vi "SaveQueue.vi"(0 "Program Interface in":refnum<class "Program Interface.lvclass">, 5 "error in (no error)":errorcluster) -> (14 "Program Interface out":refnum<class "Program Interface.lvclass">, 19 "error out":errorcluster)   [LabVIEW 2019, in "Program Interface.lvclass"]
uses:
  Program Interface.lvclass
  Program Interface.lvclass/Program Interface.ctl
  SavedQueue.ctl
  <vilib>/Utility/file.llb/Write Delimited Spreadsheet (string).vi
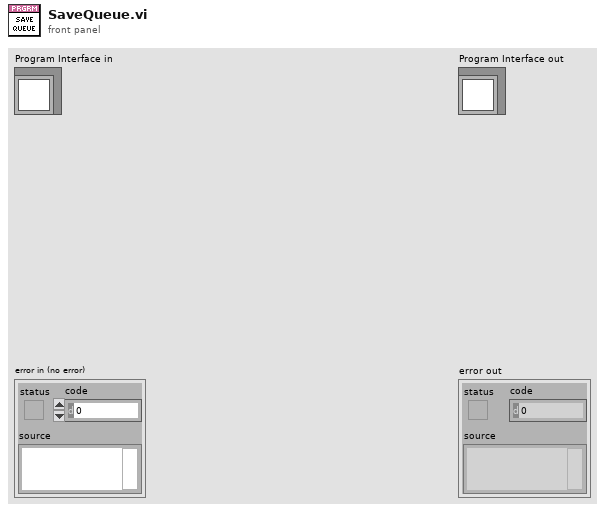
[diagram p1: front panel]
types:
  T1 = typedef "Program Interface.lvclass/SavedQueue.ctl" = cluster{"Name":string, "Programs":string[]}
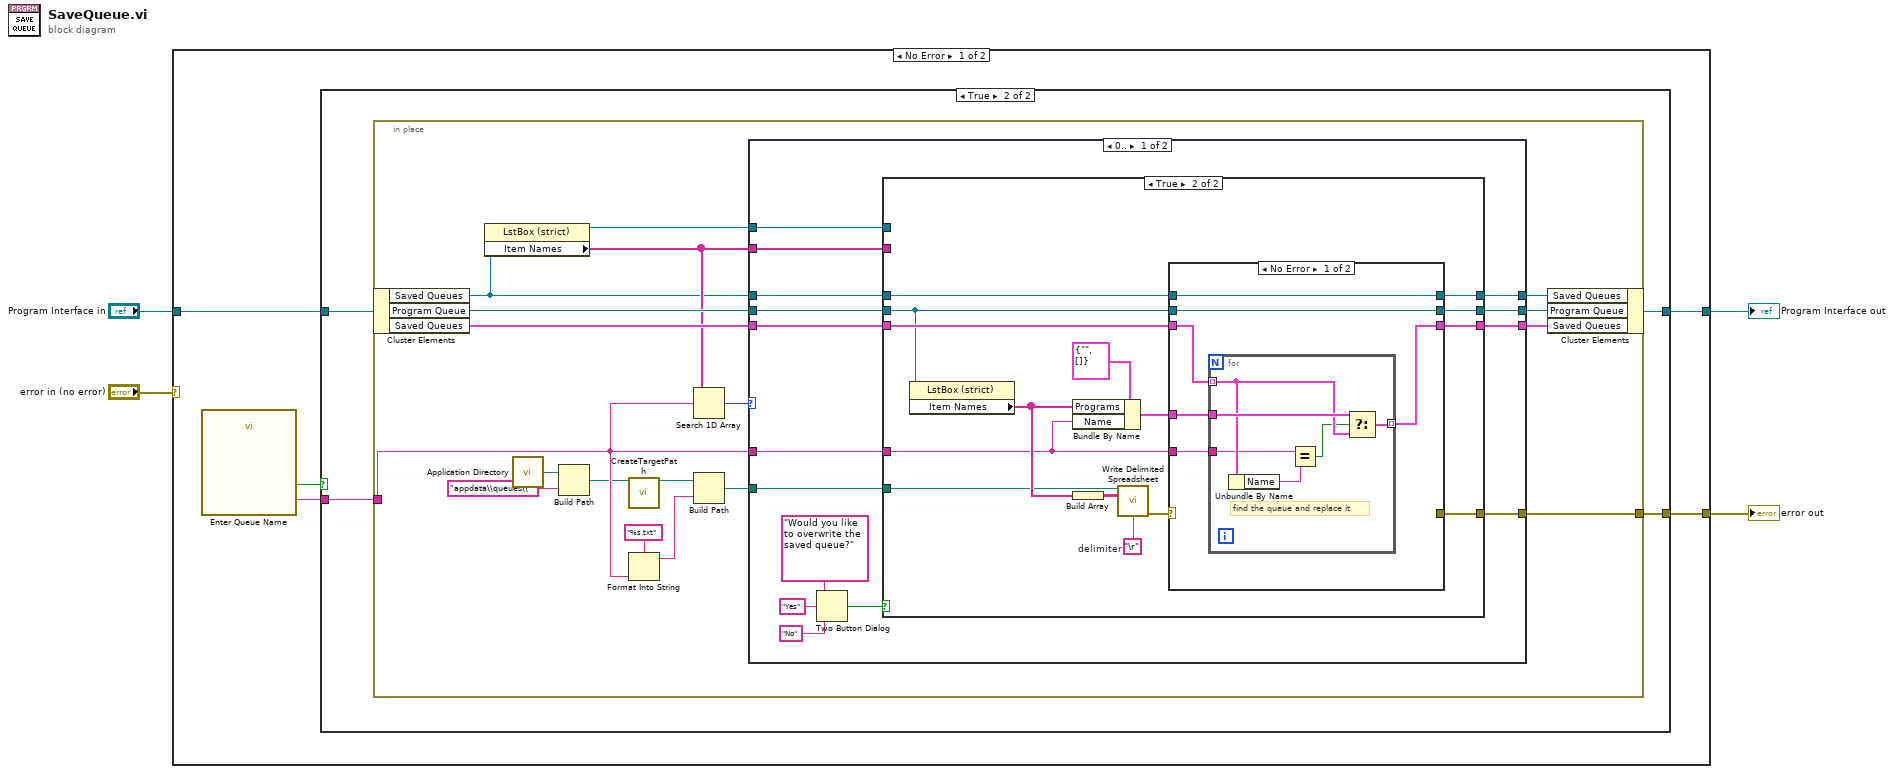
[diagram p0: block diagram]
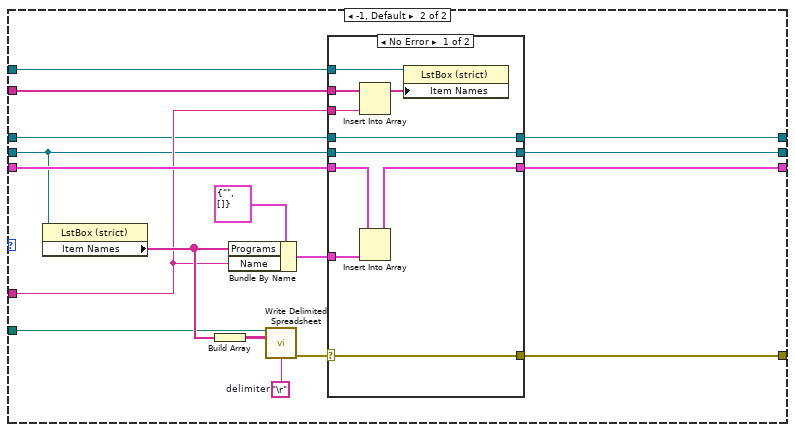
[diagram p5: hidden frame]
diagram:
  n1 = case shown="No Error" "error in (no error)" {
    selector: "error in (no error)" -> [_ w114]
    tunnel: [w9 w114] -> w3
    tunnel: [w7 w113] -> w1
    tunnel: "Program Interface in" -> [w8 w113]
    frame No Error {
      n2 = call "Enter Queue Name"() -> ("Queue Name"=w6:string, "OK"=w5:bool)  [unwired: 17 in, 1 out]
      n3 = case shown="True" w5 {
        tunnel: [_ w14] -> w9
        tunnel: w8 -> [w10 w13]
        tunnel: [w10 w12] -> w7
        tunnel: w6 -> [_ w11]
        frame False {
        }
        frame True {
          n4 = in-place {
            in-place-border: [w29] -> w14
            in-place-border: w11 -> [w26]
            n5 = in-place-cluster #1(w13) -> ("Saved Queues"=w25:refnum<vi>, "Program Queue"=w32:refnum<vi>, "Saved Queues"=w31:T1[])
            n6 = property class="LstBox (strict)"(reference=w25) -> (reference out=w28:refnum<vi>, "Item Names"=w27:string[])  [unwired: 1 in, 1 out]
            n7 = call <vilib>:"Application Directory.vi"() -> ("Application Directory"=w19:path)
            n8 = Build Path(base path=w19, name or relative path="appdata\\queues\\") -> (appended path=w20:path)
            n9 = call "CreateTargetPath.vi"("Target Path In"=w20) -> ("Target Path Out"=w21:path)  [unwired: 17 in, 1 out]
            n10 = Format Into String(format string="%s.txt", w26) -> (resulting string=w22:string)  [unwired: 2 in, 1 out]
            n11 = Search 1D Array(1D array=w27, element=w26) -> (index of element=w15:i32)  [unwired: 1 in]
            n12 = Build Path(base path=w21, name or relative path=w22) -> (appended path=w16:path)
            n13 = case shown="0.." w15 {
              tunnel: w32 -> [w41 w85]
              tunnel: w31 -> [w47 w96]
              tunnel: [w46 w92] -> w30
              tunnel: [w39 w83] -> w29
              tunnel: w28 -> [w45 w91]
              tunnel: w27 -> [w44 w90]
              tunnel: w26 -> [w37 w89]
              tunnel: w25 -> [w43 w87]
              tunnel: [w42 w86] -> w24
              tunnel: [w40 w84] -> w23
              tunnel: w16 -> [w38 w82]
              frame 0.. {
                n14 = Two Button Dialog(message="Would you like to overwrite the saved queue?" ("T button name (\"OK\")"), 1:"No" ("T button name (\"OK\")"), 2:"Yes" ("T button name (\"OK\")")) -> (T button?=w33:bool)
                n15 = case shown="True" w33 {
                  tunnel: w47 -> [w48 w63]
                  tunnel: [w48 w59] -> w46
                  tunnel: w45 -> [_ _]
                  tunnel: w44 -> [_ _]
                  tunnel: w43 -> [w50 w57]
                  tunnel: [w50 w56] -> w42
                  tunnel: w41 -> [w49 w55]
                  tunnel: [w49 w54] -> w40
                  tunnel: [_ w53] -> w39
                  tunnel: w38 -> [_ w52]
                  tunnel: w37 -> [_ w51]
                  frame False {
                  }
                  frame True {
                    w64 = "\r"  # delimiter
                    n16 = property class="LstBox (strict)"(reference=w55) -> ("Item Names"=w61:string[])  [unwired: 1 in, 2 out]
                    n17 = Bundle By Name(cluster=T1 {"Name"="", "Programs"=[]} ("Saved Queue"), "Programs"=w61, "Name"=w51) -> (w60:T1)
                    n18 = Build Array(w61) -> (w65:string[][])
                    n19 = call-poly <vilib>:"Write Delimited Spreadsheet.vi"("file path (dialog if empty)"=w52, "2D data"=w65, "delimiter (\\t)"=w64) -> ("error out"=w58:errorcluster)  [unwired: 11 in, 1 out]
                    n20 = case shown="No Error" w58 {
                      selector: w58 -> [_ w78]
                      tunnel: w63 -> [w69 w79]
                      tunnel: w60 -> [w67 _]
                      tunnel: [w66 w79] -> w59
                      tunnel: w57 -> [w71 w81]
                      tunnel: [w71 w81] -> w56
                      tunnel: w55 -> [w70 w80]
                      tunnel: [w70 w80] -> w54
                      tunnel: [_ w78] -> w53
                      tunnel: w51 -> [w68 _]
                      frame No Error {
                        n21 = for {
                          tunnel: w69 -> [w76] mode=indexing
                          tunnel: w68 -> [w74]
                          tunnel: w67 -> [w77]
                          tunnel: [w75] -> w66 mode=indexing
                          # "find the queue and replace it"
                          n22 = Unbundle By Name(w76) -> ("Name"=w73:string)
                          n23 = Equal?(x=w74, y=w73) -> (x = y?=w72:bool)
                          n24 = Select(t=w77, s=w72, f=w76) -> (s? t:f=w75:T1)
                        }
                      }
                      frame Error {
                      }
                    }
                  }
                }
              }
              frame -1, Default {
                w97 = "\r"  # delimiter
                n25 = property class="LstBox (strict)"(reference=w85) -> ("Item Names"=w94:string[])  [unwired: 1 in, 2 out]
                n26 = Build Array(w94) -> (w98:string[][])
                n27 = Bundle By Name(cluster=T1 {"Name"="", "Programs"=[]} ("Saved Queue"), "Programs"=w94, "Name"=w89) -> (w93:T1)
                n28 = call-poly <vilib>:"Write Delimited Spreadsheet.vi"("file path (dialog if empty)"=w82, "2D data"=w98, "delimiter (\\t)"=w97) -> ("error out"=w88:errorcluster)  [unwired: 11 in, 1 out]
                n29 = case shown="No Error" w88 {
                  selector: w88 -> [w99 w109]
                  tunnel: w96 -> [w108 w110]
                  tunnel: w93 -> [w107 _]
                  tunnel: [w106 w110] -> w92
                  tunnel: w91 -> [w105 _]
                  tunnel: w90 -> [w103 _]
                  tunnel: w89 -> [w102 _]
                  tunnel: w87 -> [w101 w112]
                  tunnel: [w101 w112] -> w86
                  tunnel: w85 -> [w100 w111]
                  tunnel: [w100 w111] -> w84
                  tunnel: [w99 w109] -> w83
                  frame No Error {
                    n30 = Insert Into Array(array=w103, new element=w102) -> (w104:string[])  [unwired: 1 in]
                    n31 = Insert Into Array(array=w108, new element=w107) -> (w106:T1[])  [unwired: 1 in]
                    n32 = property class="LstBox (strict)"(reference=w105, "Item Names"=w104) -> ()  [unwired: 1 in, 2 out]
                  }
                  frame Error {
                  }
                }
              }
            }
            n33 = in-place-cluster #1("Saved Queues"=w24, "Program Queue"=w23, "Saved Queues"=w30) -> (w12:refnum<class "Program Interface.lvclass">)
          }
        }
      }
    }
    frame Error {
    }
  }
  "error out" <- w3
  "Program Interface out" <- w1
